vi "SetTension.vi"(0 "level":dbl min=-505.0 max=505.0 step=1.0 format="%^.2e", 1 "compliance limit":dbl=0.025 step=1.0 format="%^.2e", 2 "range":dbl min=-505.0 max=505.0 step=1.0 format="%^.2e") -> ()   [LabVIEW 2014]
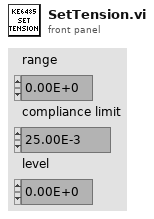
[diagram p1: front panel]
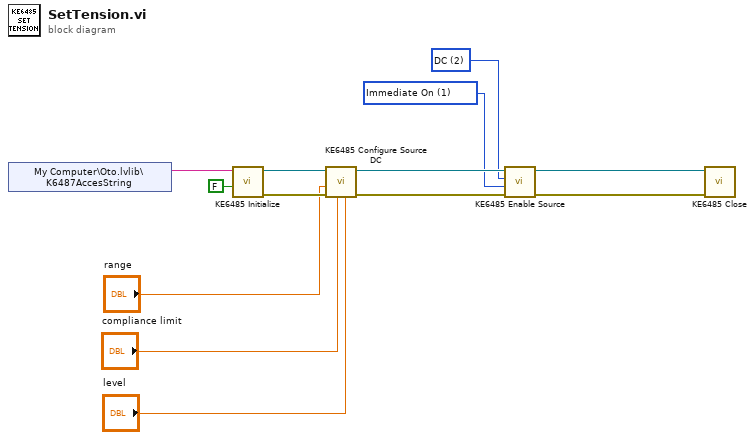
[diagram p0: block diagram]
diagram:
  w3 = 1 items=["Immediate On"=1, "Immediate Off"=2, "Immediate Standby"=4, "Auto Sync Enabled"=65536, "Auto Sync Disabled"=131072] ("output action")
  w4 = 2 items=["Bias"=1, "DC"=2, "Ramp"=4] ("generator")
  n1 = shared-variable "My Computer\\Oto.lvlib\\K6487AccesString"() -> (w2:string)  [unwired: 1 in, 1 out]
  n2 = call <instrlib>:"KE6485 Initialize.vi"("reset device"=FALSE, "resource name"=w2) -> ("error out"=w8:errorcluster, "instrument handle out"=w13:refnum<k15>)  [unwired: 8 in]
  n3 = call <instrlib>:"KE6485 Configure Source DC.vi"("level"="level", "compliance limit"="compliance limit", "error in (no error)"=w8, "range"="range", "instrument handle"=w13) -> ("error out"=w9:errorcluster, "instrument handle out"=w12:refnum<k15>)  [unwired: 5 in]
  n4 = call <instrlib>:"KE6485 Enable Source.vi"("error in (no error)"=w9, "output action"=w3, "generator"=w4, "instrument handle"=w12) -> ("error out"=w10:errorcluster, "instrument handle out"=w11:refnum<k15>)  [unwired: 6 in]
  n5 = call <instrlib>:"KE6485 Close.vi"("error in (no error)"=w10, "instrument handle"=w11) -> ()  [unwired: 9 in, 1 out]
